vi "RunTest.vi"(8 "error in":errorcluster, 11 "Prueba31 in":refnum<class "Prueba03.lvclass">) -> (0 "error out":errorcluster, 2 "Resultado":string, 3 "Prueba31 out":refnum<class "Prueba03.lvclass">)   [LabVIEW 2019, in "Prueba03.lvclass"]
uses:
  Prueba03.lvclass
  Prueba03.lvclass/Prueba03.ctl
  <vilib>/Utility/miscctls.llb/LVRowAndColumnTypeDef.ctl
  QMH/Message Queue/Enqueue Message (Single).vi
  <vilib>/Utility/error.llb/Error Cluster From Error Code.vi
  RerenceAllControlsToolkit/_get control reference by name.vi
  <vilib>/ErrorRing/Error Ring.xnode
  QMH/Message Queue/Message Queue.lvlib
  QMH/User Event - Stop/User Event - Stop.lvlib
panel:
  in  "Tab":enum32{"externo", "interno"}(tab)
  out "Pict RingB_Ext":u16(ring)
  out "curva_referencia_Ext":dbl
  in  "cb_frec_Ext":string(combo)="63"
  in  "boton_generar_Ext":bool
  out "cumple_Ext":bool
  out "no_cumple_Ext":bool
  in  "seguir_Ext":bool
  out "voltaje_Ext":dbl format="%_3f"
  out "frecuencia_Ext":dbl format="%.2f"
  out "tipo generador_Ext":string
  out "Pict RingA_Ext":u16(ring)
  in  "Tabla_Ext":string[][](table)=[["63"], ["125"], ["250"], ["500"], ["1000"], ["2000"], ["4000"], ["8000"]]
  out "cumple_Int":bool
  out "no_cumple_Int":bool
  in  "seguir_Int":bool
  out "tipo generador_Int":string
  out "Pict RingA_Int":u16(ring)
  out "Pict RingB_Int":u16(ring)
  in  "Tabla_Int":string[][](table)
  # "Vienen de base de datos\nambos\ncambiar a numerico indicador"
  # "Cumple"
  # "No Cumple"
  # "Ponderación C"
  # "Curva de Referencia"
  # "Frecuencia"
  # "3. Ensayo con ponderación frecuencial C con señales acústicas. IEC 61672-3:2006 Cláusula 11"
  # "Monitoreo"
  # "Frecuencia"
  # "Hz"
  # "Voltaje"
  # "V"
  # "Cumple"
  # "No Cumple"
  # "Ponderación C"
  # "3. Ensayo con ponderación frecuencial C con señales acústicas. IEC 61672-3:2006 Cláusula 11"
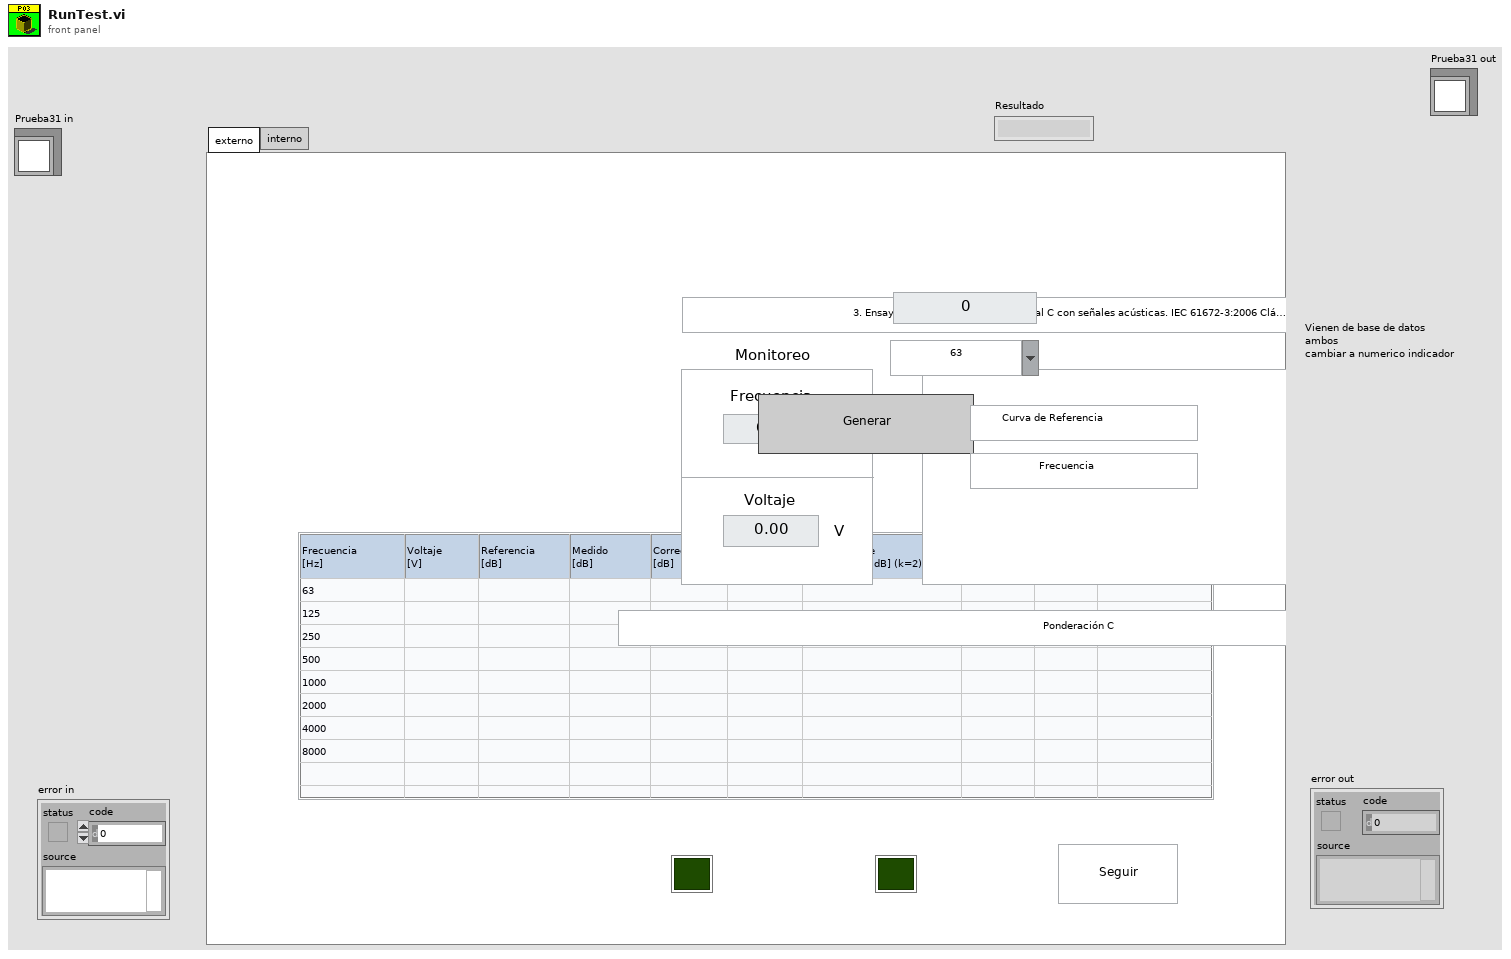
[diagram p1: front panel]
types:
  T1 = typedef "Message Queue.lvlib/All Message Queues.ctl" = cluster{"MHL":refnum<queue>, "Inst_CNT90":refnum<queue>, "Inst_DS360":refnum<queue>, "Inst_Keithley2002":refnum<queue>, "Inst_DAQ":refnum<queue>, "BD":refnum<queue>, "Pistofono":refnum<queue>, "Nexus":refnum<queue>}
  T2 = typedef "LVRowAndColumnTypeDef.ctl" = cluster{"Row":i32, "Column":i32}
  T3 = cluster{"ControlName":string, "ControlReference":refnum<vi>}[]
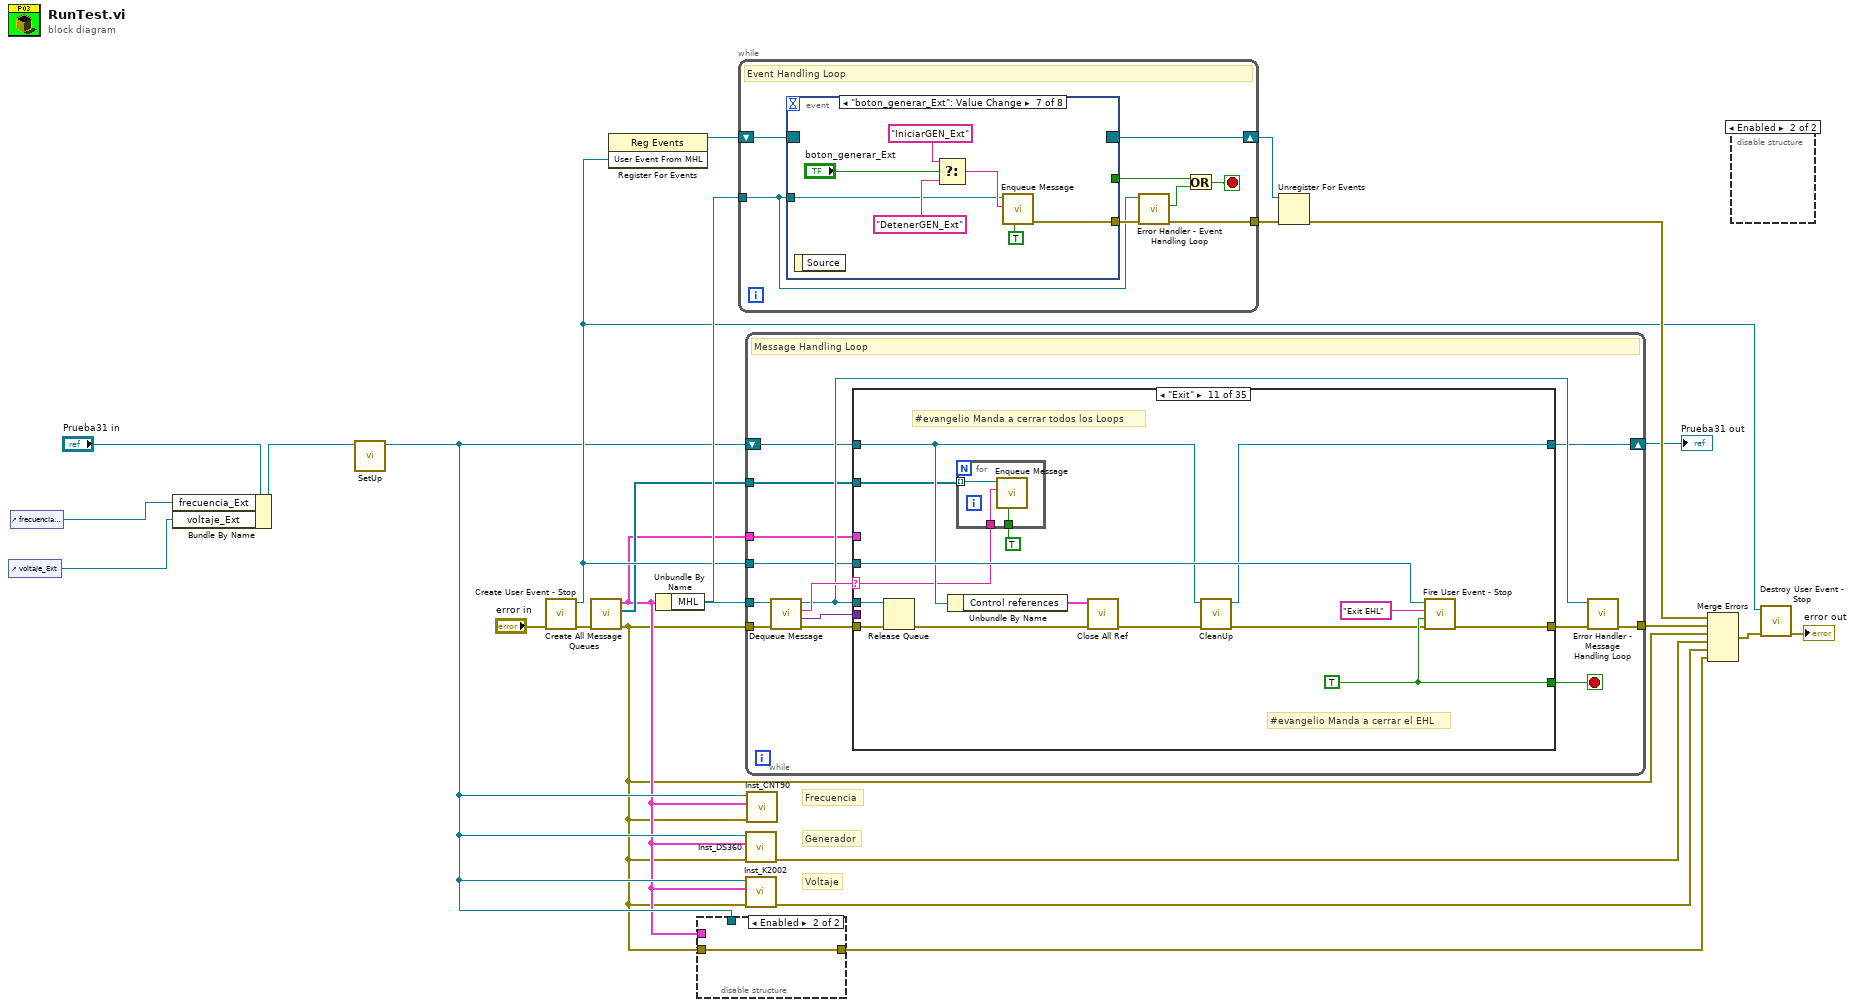
[diagram p0: block diagram]
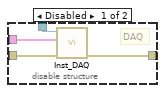
[diagram p2: hidden frame]
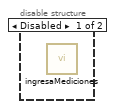
[diagram p3: hidden frame]
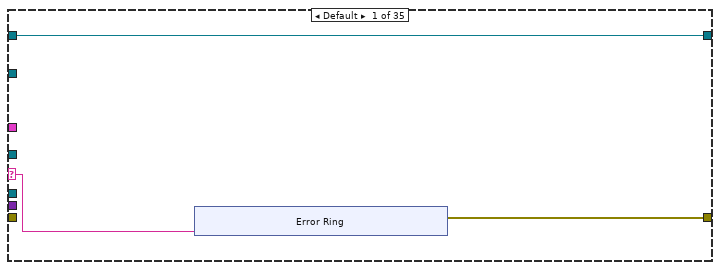
[diagram p4: hidden frame]
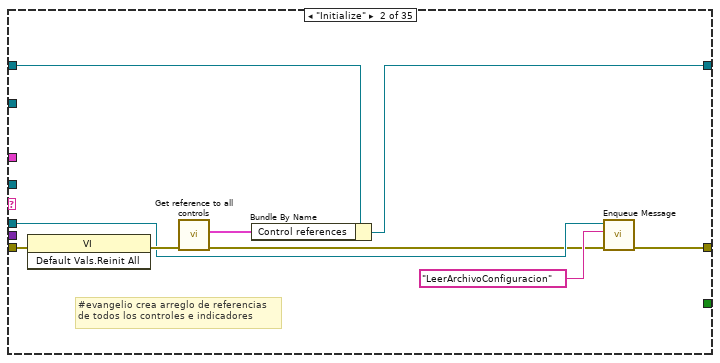
[diagram p5: hidden frame]
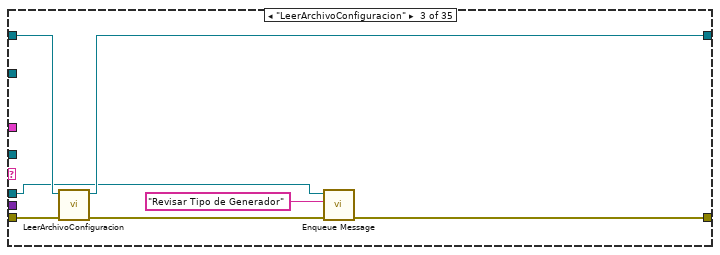
[diagram p6: hidden frame]
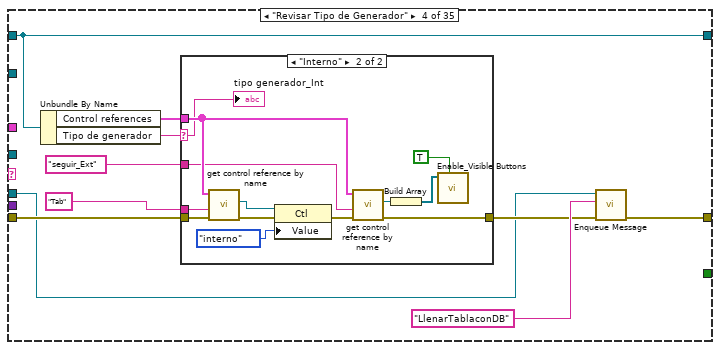
[diagram p7: hidden frame]
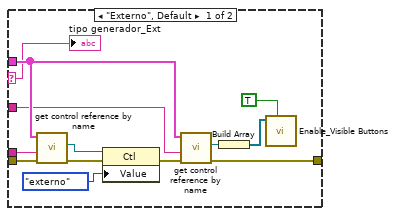
[diagram p8: hidden frame]
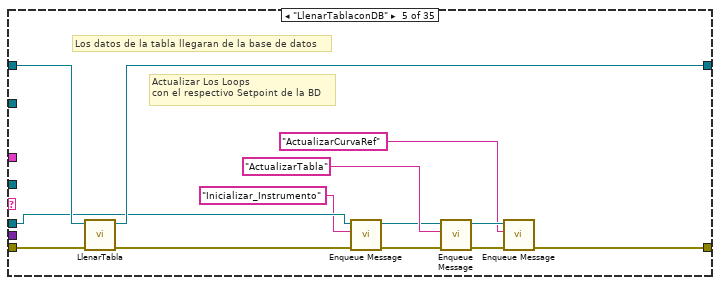
[diagram p9: hidden frame]
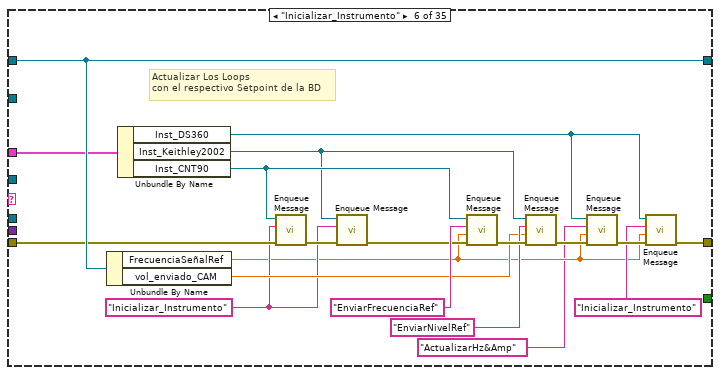
[diagram p10: hidden frame]
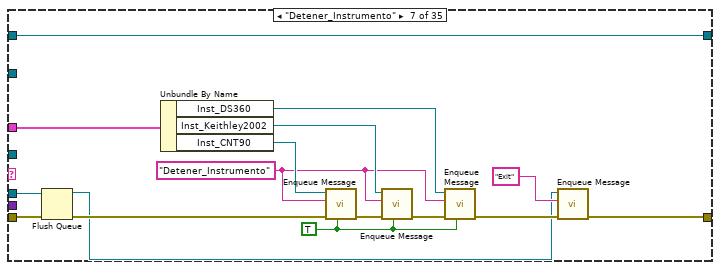
[diagram p11: hidden frame]
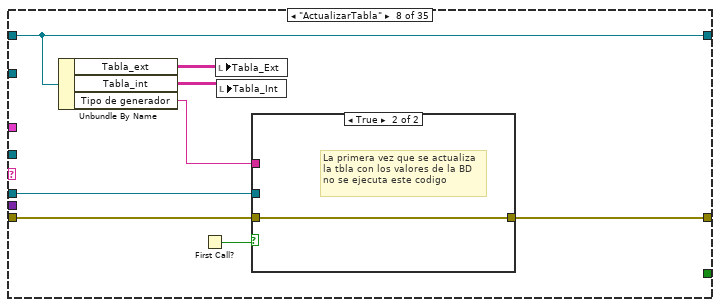
[diagram p12: hidden frame]
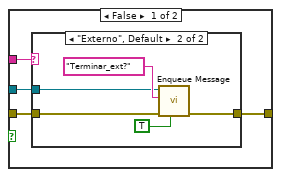
[diagram p13: hidden frame]
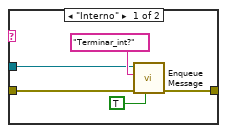
[diagram p14: hidden frame]
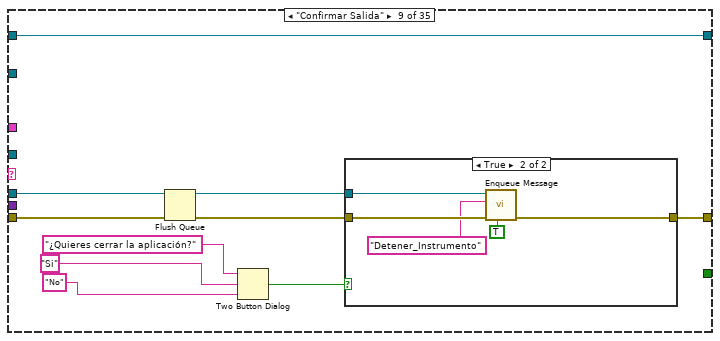
[diagram p15: hidden frame]
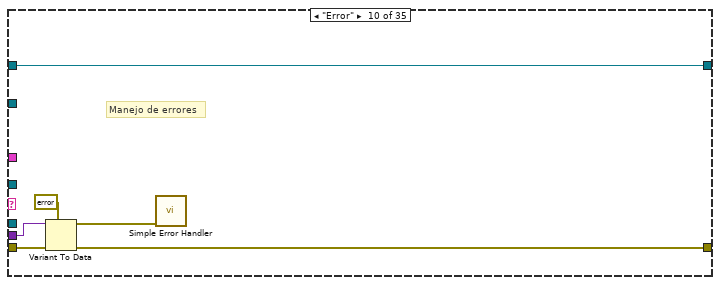
[diagram p17: hidden frame]
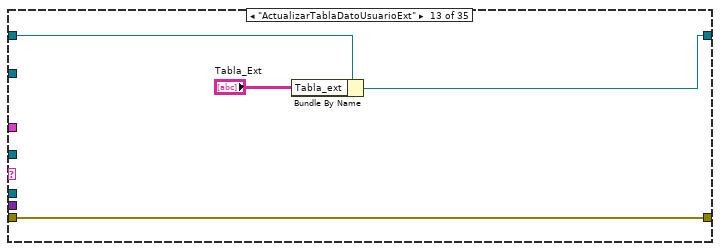
[diagram p19: hidden frame]
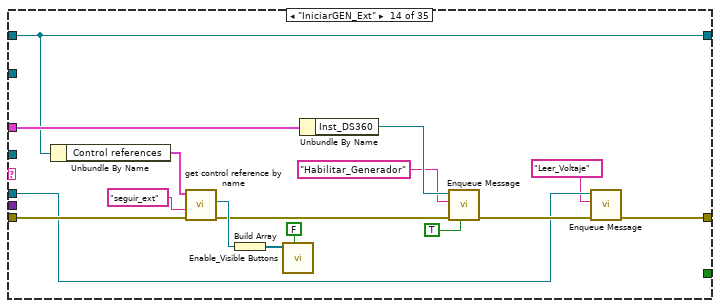
[diagram p20: hidden frame]
diagram:
  # "Voltaje"
  # "Generador"
  # "Frecuencia"
  n1 = control-ref of="voltaje_Ext"() -> (w1:refnum<vi>)
  n2 = control-ref of="frecuencia_Ext"() -> (w2:refnum<vi>)
  n3 = Bundle By Name(cluster="Prueba31 in", "frecuencia_Ext"=w2, "voltaje_Ext"=w1) -> (w3:refnum<class "Prueba03.lvclass">)
  n4 = call-dynamic "SetUp.vi"("Prueba03 in"=w3) -> ("Prueba03 out"=w6:refnum<class "Prueba03.lvclass">)  [unwired: 9 in, 1 out]
  n5 = call "Create User Event - Stop.vi"("error in (no error)"="error in") -> ("error out"=w20:errorcluster, "User Event From MHL"=w14:refnum<user-event>)  [unwired: 9 in]
  n6 = call "Create All Message Queues.vi"("error in (no error)"=w20) -> ("error out"=w4:errorcluster, "PL Queues Array"=w9:refnum<queue>[], "All Message Queues out"=w5:T1)  [unwired: 8 in]
  n7 = register-events(w14) -> (reference out=w23:refnum<event-registration>)  [unwired: 2 in, 1 out]
  n8 = Unbundle By Name(w5) -> ("MHL"=w19:refnum<queue>)
  n9 = disable-structure shown="Enabled" {
    disable-tunnel: w5 -> [w27 _]
    disable-tunnel: w4 -> [w26 w28]
    disable-tunnel: [w25 w28] -> w8
    disable-tunnel: w6 -> [w24 _]
    frame Disabled {
      # "DAQ"
      n10 = call "Inst_DAQ.vi"("error in"=w26, "All Message Queues in"=w27, "Prueba31 in"=w24) -> ("error out"=w25:errorcluster)  [unwired: 8 in]
    }
    frame Enabled {
    }
  }
  n11 = while {
    tunnel: w19 -> [w29]
    tunnel: [w33] -> w22
    shift-right: [w35] -> w21
    shift-left: w23 -> [w36]
    stop <- w30 stop-if-true
    # "Event Handling Loop"
    n12 = event shown="[6] \"boton_generar_Ext\": Value Change" {
      selector: w36 -> [_ _ _ _ _ _ _ _]
      dyn-events: [_ _ _ _ _ _ _ _] -> w35
      timeout: _ -> [_ _ _ _ _ _ _ _]
      tunnel: w29 -> [w39 _ w50 w53 w59 w63 w70 w77]
      tunnel: [w40 _ w47 w54 w61 w68 w75 w78] -> w34
      tunnel: [_ w41 _ _ _ _ _ _] -> w31
      event Panel Close? {
        w37 = TRUE
        n13 = event-data() -> ()  [unwired: 1 in, 1 out]
        n14 = call-poly "Enqueue Message.vi"("Priority Message? (F)"=w37, "Message"="Confirmar Salida", "Message Queue"=w39) -> ("error out"=w40:errorcluster)  [unwired: 7 in, 1 out]
        n15 = event-data("Discard?"=w37) -> ()  [unwired: 1 in, 1 out]
      }
      event User Event {
        n16 = event-data() -> ("User Event"=w43:string, "Event Data"=w42:variant)  [unwired: 1 in]
        n17 = case shown="\"Exit EHL\"" w43 {
          tunnel: w42 -> [_ w45]
          tunnel: [_ w44] -> w41
          frame Default {
          }
          frame "Exit EHL" {
            # "#evangelio Termina\nla ejecucion del EHL"
            n18 = Variant To Data(type=TRUE, Variant=w45) -> (data=w44:bool)  [unwired: 1 in, 1 out]
          }
        }
      }
      event "seguir_Ext": Value Change {
        n19 = event-data() -> ()  [unwired: 1 in, 1 out]
        n20 = call-poly "Enqueue Message.vi"("Priority Message? (F)"=TRUE, "Message"="Detener_Instrumento", "Message Queue"=w50) -> ("error out"=w47:errorcluster)  [unwired: 7 in, 1 out]
      }
      event "seguir_Int": Value Change {
        n21 = event-data() -> ()  [unwired: 1 in, 1 out]
        n22 = call-poly "Enqueue Message.vi"("Priority Message? (F)"=TRUE, "Message"="Exit", "Message Queue"=w53) -> ("error out"=w54:errorcluster)  [unwired: 7 in, 1 out]
      }
      event "Tabla_Ext": Value Change {
        n23 = event-data() -> ()  [unwired: 1 in, 1 out]
        n24 = property on="Tabla_Ext" class="Tbl (strict)"() -> ("Selection Start"=w55:T2)  [unwired: 2 in, 2 out]
        n25 = call-poly "Enqueue Message.vi"("Message"="ActualizarTablaDatoUsuarioExt", "Message Queue"=w59) -> ("error out"=w56:errorcluster, "dup Message Queue"=w58:refnum<queue>)  [unwired: 8 in]
        n26 = call-poly "Enqueue Message.vi"("error in (no error)"=w56, "Message Data"=w55, "Message"="Evaluacion_Ext", "Message Queue"=w58) -> ("error out"=w61:errorcluster)  [unwired: 6 in, 1 out]
      }
      event "Tabla_Int": Value Change {
        n27 = event-data() -> ()  [unwired: 1 in, 2 out]
        n28 = property on="Tabla_Int" class="Tbl (strict)"() -> ("Selection Start"=w66:T2)  [unwired: 2 in, 2 out]
        n29 = call-poly "Enqueue Message.vi"("Message"="ActualizarTablaDatoUsuarioInt", "Message Queue"=w63) -> ("error out"=w65:errorcluster, "dup Message Queue"=w64:refnum<queue>)  [unwired: 8 in]
        n30 = call-poly "Enqueue Message.vi"("error in (no error)"=w65, "Message Data"=w66, "Message"="Evaluacion_Int", "Message Queue"=w64) -> ("error out"=w68:errorcluster)  [unwired: 6 in, 1 out]
      }
      event "boton_generar_Ext": Value Change {
        n31 = event-data() -> ()  [unwired: 1 in, 1 out]
        n32 = Select(t="IniciarGEN_Ext" ("Message"), s="boton_generar_Ext", f="DetenerGEN_Ext" ("Message")) -> (s? t:f=w73:string)
        n33 = call-poly "Enqueue Message.vi"("Priority Message? (F)"=TRUE, "Message"=w73, "Message Queue"=w70) -> ("error out"=w75:errorcluster)  [unwired: 7 in, 1 out]
      }
      event "cb_frec_Ext": Value Change {
        (unwired) "ActualizarCurvaRef" ("Message")
        n34 = event-data() -> ()  [unwired: 1 in, 1 out]
        n35 = call-poly "Enqueue Message.vi"("Message"="NuevoValorFrecuencia", "Message Queue"=w77) -> ("error out"=w78:errorcluster)  [unwired: 8 in, 1 out]
      }
    }
    n36 = call "Error Handler - Event Handling Loop.vi"("error in (no error)"=w34, "Message Queue"=w29) -> ("dup error in"=w33:errorcluster, "Error?"=w32:bool)  [unwired: 7 in, 1 out]
    n37 = Or(x=w31, y=w32) -> (x .or. y?=w30:bool)
  }
  n38 = while {
    tunnel: w4 -> [w92]
    tunnel: w19 -> [w91]
    tunnel: [w85] -> w17
    shift-right: [w83] -> w15
    shift-left: w6 -> [w84]
    tunnel: w5 -> [w81]
    tunnel: w14 -> [w80]
    tunnel: w9 -> [w79]
    stop <- w82 stop-if-true
    # "Message Handling Loop"
    n39 = call "Dequeue Message.vi"("error in (no error)"=w92, "Message Queue"=w91) -> ("error out"=w88:errorcluster, "Message Data"=w89:variant, "Message"=w90:string, "dup Message Queue"=w87:refnum<queue>)  [unwired: 6 in]
    n40 = case shown="\"Exit\"" w90 {
      selector: w90 -> [w94 _ _ _ _ _ _ _ _ _ w249 _ _ _ _ _ _ _ _ _ w368 w377 _ _ _ _ _ _ _ _ _ _ _ _ _]
      tunnel: w87 -> [_ w106 w113 w119 w157 _ w190 w205 w226 _ w260 _ _ w272 w287 w297 w322 _ _ _ w363 _ w389 w406 _ w436 _ w458 w470 _ _ w484 w501 _ _]
      tunnel: w89 -> [_ _ _ _ _ _ _ _ _ w242 _ _ _ _ _ _ _ w337 w345 w348 w374 w384 w401 _ _ _ _ _ _ _ _ w496 _ _ _]
      tunnel: w88 -> [_ w111 w118 w125 w167 w178 w194 w206 w233 w243 w259 w266 w270 w279 w290 w300 w323 w338 w346 w349 w375 w385 w402 w415 w431 w440 w455 w465 w474 w477 w481 w497 w510 w529 w534]
      tunnel: [w93 w107 w114 w120 w160 w172 w189 w204 w232 w244 w257 w266 w270 w285 w289 w299 w314 w339 w347 w350 w372 w381 w393 w409 w431 w437 w451 w463 w473 w477 w481 w487 w504 w529 w534] -> w86
      tunnel: w84 -> [w95 w109 w117 w124 w166 w186 w201 w209 w234 w246 w250 w265 w268 w280 w294 w304 w328 w340 w343 w351 w376 w386 w397 w411 w427 w439 w454 w466 w475 w476 w479 w492 w506 w525 w533]
      tunnel: [w95 w108 w116 w124 w163 w186 w201 w209 w234 w246 w251 w265 w269 w280 w294 w304 w329 w340 w344 w351 w376 w386 w404 w411 w427 w439 w454 w461 w475 w476 w480 w499 w506 w525 w533] -> w83
      tunnel: [_ _ _ _ _ _ _ _ _ _ w254 _ _ _ _ _ _ _ _ _ _ _ _ _ _ _ _ _ _ _ _ _ _ _ _] -> w82
      tunnel: w81 -> [_ _ _ _ _ w184 w192 _ _ _ _ _ _ w286 w296 w306 w316 _ _ _ w371 w379 _ _ _ _ _ _ _ _ _ _ _ _ _]
      tunnel: w80 -> [_ _ _ _ _ _ _ _ _ _ w256 _ _ _ _ _ _ _ _ _ _ _ _ _ _ _ _ _ _ _ _ _ _ _ _]
      tunnel: w79 -> [_ _ _ _ _ _ _ _ _ _ w247 _ _ _ _ _ _ _ _ _ _ _ _ _ _ _ _ _ _ _ _ _ _ _ _]
      frame Default {
        n41 = xnode "Error Ring"("parameter 0"=w94) -> ("error out"=w93:errorcluster)
      }
      frame "Initialize" {
        # "#evangelio crea arreglo de referencias\nde todos los controles e indicadores"
        n42 = invoke class="VI" method="Default Vals.Reinit All"(error in=w111) -> (error out=w110:errorcluster)  [unwired: 2 in, 2 out]
        n43 = call "Get reference to all controls.vi"("error in (no error)"=w110) -> ("error out"=w103:errorcluster, "Control references"=w104:T3)  [unwired: 5 in]
        n44 = Bundle By Name(cluster=w109, "Control references"=w104) -> (w108:refnum<class "Prueba03.lvclass">)
        n45 = call-poly "Enqueue Message.vi"("error in (no error)"=w103, "Message"="LeerArchivoConfiguracion", "Message Queue"=w106) -> ("error out"=w107:errorcluster)  [unwired: 7 in, 1 out]
      }
      frame "LeerArchivoConfiguracion" {
        n46 = call "LeerArchivoConfiguracion.vi"("error in"=w118, "Prueba31 in"=w117) -> ("error out"=w115:errorcluster, "Prueba31 out"=w116:refnum<class "Prueba03.lvclass">)  [unwired: 8 in]
        n47 = call-poly "Enqueue Message.vi"("error in (no error)"=w115, "Message"="Revisar Tipo de Generador", "Message Queue"=w113) -> ("error out"=w114:errorcluster)  [unwired: 7 in, 1 out]
      }
      frame "Revisar Tipo de Generador" {
        n48 = Unbundle By Name(w124) -> ("Control references"=w127:T3, "Tipo de generador"=w128:string)
        n49 = case shown="\"Interno\"" w128 {
          selector: w128 -> [w129 w142]
          tunnel: w125 -> [w141 w154]
          tunnel: w127 -> [w136 w149]
          tunnel: "Tab" -> [w140 w153]
          tunnel: "seguir_Ext" -> [w134 w147]
          tunnel: [w131 w144] -> w121
          frame "Externo", Default {
            n50 = call-poly "get control reference by name.vi"("error in (no error)"=w141, "Control name"=w140, "Control references"=w136) -> ("error out"=w138:errorcluster, "Ctl Refnum"=w139:refnum<vi>)  [unwired: 3 in]
            n51 = property class="Ctl"(reference=w139, error in=w138, "Value"=enum32{"externo", "interno"}."externo" ("Tab Control")) -> (error out=w135:errorcluster)  [unwired: 1 out]
            n52 = call-poly "get control reference by name.vi"("error in (no error)"=w135, "Control name"=w134, "Control references"=w136) -> ("error out"=w131:errorcluster, "Ctl Refnum"=w133:refnum<vi>)  [unwired: 3 in]
            n53 = Build Array(w133) -> (w132:refnum<vi>[])
            n54 = call "Enable_Visible Buttons.vi"("Enable? (T)"=TRUE, "Controls Ref Array"=w132) -> ()  [unwired: 10 in]
            "tipo generador_Ext" <- w129
          }
          frame "Interno" {
            n55 = call-poly "get control reference by name.vi"("error in (no error)"=w154, "Control name"=w153, "Control references"=w149) -> ("error out"=w151:errorcluster, "Ctl Refnum"=w152:refnum<vi>)  [unwired: 3 in]
            n56 = property class="Ctl"(reference=w152, error in=w151, "Value"=enum32{"externo", "interno"}."interno" ("Tab Control")) -> (error out=w148:errorcluster)  [unwired: 1 out]
            n57 = call-poly "get control reference by name.vi"("error in (no error)"=w148, "Control name"=w147, "Control references"=w149) -> ("error out"=w144:errorcluster, "Ctl Refnum"=w146:refnum<vi>)  [unwired: 3 in]
            n58 = Build Array(w146) -> (w145:refnum<vi>[])
            n59 = call "Enable_Visible Buttons.vi"("Enable? (T)"=TRUE, "Controls Ref Array"=w145) -> ()  [unwired: 10 in]
            "tipo generador_Int" <- w142
          }
        }
        n60 = call-poly "Enqueue Message.vi"("error in (no error)"=w121, "Message"="LlenarTablaconDB", "Message Queue"=w119) -> ("error out"=w120:errorcluster)  [unwired: 7 in, 1 out]
      }
      frame "LlenarTablaconDB" {
        # "Actualizar Los Loops\ncon el respectivo Setpoint de la BD"
        # "Los datos de la tabla llegaran de la base de datos"
        n61 = call "LlenarTabla.vi"("error in (no error)"=w167, "Prueba32 in"=w166) -> ("error out"=w165:errorcluster, "Prueba32 out"=w163:refnum<class "Prueba03.lvclass">)  [unwired: 8 in]
        n62 = call-poly "Enqueue Message.vi"("error in (no error)"=w165, "Message"="Inicializar_Instrumento", "Message Queue"=w157) -> ("error out"=w158:errorcluster, "dup Message Queue"=w156:refnum<queue>)  [unwired: 7 in]
        n63 = call-poly "Enqueue Message.vi"("error in (no error)"=w158, "Message"="ActualizarTabla", "Message Queue"=w156) -> ("error out"=w161:errorcluster, "dup Message Queue"=w162:refnum<queue>)  [unwired: 7 in]
        n64 = call-poly "Enqueue Message.vi"("error in (no error)"=w161, "Message"="ActualizarCurvaRef", "Message Queue"=w162) -> ("error out"=w160:errorcluster)  [unwired: 7 in, 1 out]
      }
      frame "Inicializar_Instrumento" {
        w174 = "Inicializar_Instrumento" ("Message")
        # "Actualizar Los Loops\ncon el respectivo Setpoint de la BD"
        n65 = Unbundle By Name(w186) -> ("FrecuenciaSeñalRef"=w169:dbl, "vol_enviado_CAM"=w181:dbl)
        n66 = Unbundle By Name(w184) -> ("Inst_DS360"=w171:refnum<queue>, "Inst_Keithley2002"=w175:refnum<queue>, "Inst_CNT90"=w179:refnum<queue>)
        n67 = call-poly "Enqueue Message.vi"("error in (no error)"=w178, "Message"=w174, "Message Queue"=w179) -> ("error out"=w177:errorcluster)  [unwired: 7 in, 1 out]
        n68 = call-poly "Enqueue Message.vi"("error in (no error)"=w177, "Message"=w174, "Message Queue"=w175) -> ("error out"=w176:errorcluster)  [unwired: 7 in, 1 out]
        n69 = call-poly "Enqueue Message.vi"("error in (no error)"=w176, "Message Data"=w169, "Message"="EnviarFrecuenciaRef", "Message Queue"=w179) -> ("error out"=w185:errorcluster)  [unwired: 6 in, 1 out]
        n70 = call-poly "Enqueue Message.vi"("error in (no error)"=w185, "Message Data"=w181, "Message"="EnviarNivelRef", "Message Queue"=w175) -> ("error out"=w180:errorcluster)  [unwired: 6 in, 1 out]
        n71 = call-poly "Enqueue Message.vi"("error in (no error)"=w180, "Message Data"=w169, "Message"="ActualizarHz&Amp", "Message Queue"=w171) -> ("error out"=w173:errorcluster)  [unwired: 6 in, 1 out]
        n72 = call-poly "Enqueue Message.vi"("error in (no error)"=w173, "Message Data"=w169, "Message"="Inicializar_Instrumento", "Message Queue"=w171) -> ("error out"=w172:errorcluster)  [unwired: 6 in, 1 out]
      }
      frame "Detener_Instrumento" {
        w195 = TRUE ("Priority Message? (F)")
        w196 = "Detener_Instrumento" ("Message")
        n73 = Flush Queue(queue=w190, error in (no error)=w194) -> (queue out=w187:refnum<queue>, error out=w191:errorcluster)  [unwired: 1 out]
        n74 = Unbundle By Name(w192) -> ("Inst_DS360"=w197:refnum<queue>, "Inst_Keithley2002"=w198:refnum<queue>, "Inst_CNT90"=w200:refnum<queue>)
        n75 = call-poly "Enqueue Message.vi"("Priority Message? (F)"=w195, "error in (no error)"=w191, "Message"=w196, "Message Queue"=w200) -> ("error out"=w199:errorcluster)  [unwired: 6 in, 1 out]
        n76 = call-poly "Enqueue Message.vi"("Priority Message? (F)"=w195, "error in (no error)"=w199, "Message"=w196, "Message Queue"=w198) -> ("error out"=w193:errorcluster)  [unwired: 6 in, 1 out]
        n77 = call-poly "Enqueue Message.vi"("Priority Message? (F)"=w195, "Message"=w196, "Message Queue"=w197) -> ()  [unwired: 7 in, 2 out]
        n78 = call-poly "Enqueue Message.vi"("error in (no error)"=w193, "Message"="Exit", "Message Queue"=w187) -> ("error out"=w189:errorcluster)  [unwired: 7 in, 1 out]
      }
      frame "ActualizarTabla" {
        n79 = Unbundle By Name(w209) -> ("Tabla_ext"=w208:string[][], "Tabla_int"=w207:string[][], "Tipo de generador"=w203:string)
        n80 = First Call?() -> (First Call?: T/F=w202:bool)
        n81 = local write "Tabla_Ext"(w208) -> ()
        n82 = local write "Tabla_Int"(w207) -> ()
        n83 = case shown="True" w202 {
          tunnel: w206 -> [w213 w224]
          tunnel: w205 -> [w212 _]
          tunnel: [w211 w224] -> w204
          tunnel: w203 -> [w210 _]
          frame False {
            n84 = case shown="\"Externo\", Default" w210 {
              tunnel: w213 -> [w216 w222]
              tunnel: w212 -> [w217 w221]
              tunnel: [w215 w220] -> w211
              frame "Interno" {
                n85 = call-poly "Enqueue Message.vi"("Priority Message? (F)"=TRUE, "error in (no error)"=w216, "Message"="Terminar_int?", "Message Queue"=w217) -> ("error out"=w215:errorcluster)  [unwired: 6 in, 1 out]
              }
              frame "Externo", Default {
                n86 = call-poly "Enqueue Message.vi"("Priority Message? (F)"=TRUE, "error in (no error)"=w222, "Message"="Terminar_ext?", "Message Queue"=w221) -> ("error out"=w220:errorcluster)  [unwired: 6 in, 1 out]
              }
            }
          }
          frame True {
            # "La primera vez que se actualiza\nla tbla con los valores de la BD\nno se ejecuta este codigo"
          }
        }
      }
      frame "Confirmar Salida" {
        n87 = Flush Queue(queue=w226, error in (no error)=w233) -> (queue out=w225:refnum<queue>, error out=w227:errorcluster)  [unwired: 1 out]
        n88 = Two Button Dialog(message="¿Quieres cerrar la aplicación?", 1:"No" ("T button name (\"OK\")"), 2:"Si" ("T button name (\"OK\")")) -> (T button?=w228:bool)
        n89 = case shown="True" w228 {
          tunnel: w227 -> [w235 w240]
          tunnel: [w235 w237] -> w232
          tunnel: w225 -> [_ w238]
          frame False {
          }
          frame True {
            n90 = call-poly "Enqueue Message.vi"("Priority Message? (F)"=TRUE, "error in (no error)"=w240, "Message"="Detener_Instrumento", "Message Queue"=w238) -> ("error out"=w237:errorcluster)  [unwired: 6 in, 1 out]
          }
        }
      }
      frame "Error" {
        # "Manejo de errores"
        n91 = Variant To Data(error in=w243, type=errorcluster {"status"=FALSE, "code"=0, "source"=""} ("error constant"), Variant=w242) -> (data=w241:errorcluster, error out=w244:errorcluster)
        n92 = call <vilib>:"Simple Error Handler.vi"("error in (no error)"=w241) -> ()  [unwired: 4 in, 5 out]
      }
      frame "Exit" {
        w254 = TRUE
        # "#evangelio Manda a cerrar el EHL"
        # "#evangelio Manda a cerrar todos los Loops"
        n93 = Release Queue(queue=w260, error in (no error)=w259) -> (error out=w258:errorcluster)  [unwired: 1 in, 2 out]
        n94 = Unbundle By Name(w250) -> ("Control references"=w261:T3)
        n95 = for {
          tunnel: w247 -> [w264] mode=indexing
          tunnel: w249 -> [w263]
          tunnel: TRUE -> [w262]
          n96 = call-poly "Enqueue Message.vi"("Priority Message? (F)"=w262, "Message"=w263, "Message Queue"=w264) -> ()  [unwired: 7 in, 2 out]
        }
        n97 = call "Close All Ref.vi"("error in (no error)"=w258, "Control references"=w261) -> ("error out"=w253:errorcluster)  [unwired: 9 in]
        n98 = call-dynamic "CleanUp.vi"("error in (no error)"=w253, "Prueba03 in"=w250) -> ("error out"=w252:errorcluster, "Prueba03 out"=w251:refnum<class "Prueba03.lvclass">)  [unwired: 8 in]
        n99 = call "Fire User Event - Stop.vi"("error in (no error)"=w252, "Event Data"=w254, "User Event"="Exit EHL", "User Event in"=w256) -> ("error out"=w257:errorcluster)  [unwired: 7 in]
      }
      frame "---- EXT ----" {
      }
      frame "ActualizarTablaDatoUsuarioExt" {
        n100 = Bundle By Name(cluster=w268, "Tabla_ext"="Tabla_Ext") -> (w269:refnum<class "Prueba03.lvclass">)
      }
      frame "IniciarGEN_Ext" {
        n101 = Unbundle By Name(w280) -> ("Control references"=w281:T3)
        n102 = call-poly "get control reference by name.vi"("error in (no error)"=w279, "Control name"="seguir_ext", "Control references"=w281) -> ("error out"=w275:errorcluster, "Ctl Refnum"=w283:refnum<vi>)  [unwired: 3 in]
        n103 = Build Array(w283) -> (w282:refnum<vi>[])
        n104 = call "Enable_Visible Buttons.vi"("Enable? (T)"=FALSE, "Controls Ref Array"=w282) -> ()  [unwired: 10 in]
        n105 = Unbundle By Name(w286) -> ("Inst_DS360"=w277:refnum<queue>)
        n106 = call-poly "Enqueue Message.vi"("Priority Message? (F)"=TRUE, "error in (no error)"=w275, "Message"="Habilitar_Generador", "Message Queue"=w277) -> ("error out"=w274:errorcluster)  [unwired: 6 in, 1 out]
        n107 = call-poly "Enqueue Message.vi"("error in (no error)"=w274, "Message"="Leer_Voltaje", "Message Queue"=w272) -> ("error out"=w285:errorcluster)  [unwired: 7 in, 1 out]
      }
      frame "Leer_Voltaje" {
        n108 = call-poly "Enqueue Message.vi"("error in (no error)"=w290, "Message"="Leer_Frecuencia", "Message Queue"=w287) -> ("error out"=w295:errorcluster)  [unwired: 7 in, 1 out]
        n109 = Unbundle By Name(w296) -> ("Inst_Keithley2002"=w293:refnum<queue>)
        n110 = call-poly "Enqueue Message.vi"("Message"="Leer_Instrumento", "Message Queue"=w293) -> ()  [unwired: 8 in, 2 out]
        n111 = call "Time Delay"("error in (no error)"=w295, "Delay Time (s)"=1.0) -> ("error out"=w289:errorcluster)  [unwired: 9 in]
      }
      frame "Leer_Frecuencia" {
        n112 = call-poly "Enqueue Message.vi"("error in (no error)"=w300, "Message"="Leer_Voltaje", "Message Queue"=w297) -> ("error out"=w305:errorcluster)  [unwired: 7 in, 1 out]
        n113 = Unbundle By Name(w306) -> ("Inst_CNT90"=w303:refnum<queue>)
        n114 = call-poly "Enqueue Message.vi"("Message"="Leer_Instrumento", "Message Queue"=w303) -> ()  [unwired: 8 in, 2 out]
        n115 = call "Time Delay2"("error in (no error)"=w305, "Delay Time (s)"=1.0) -> ("error out"=w299:errorcluster)  [unwired: 9 in]
      }
      frame "DetenerGEN_Ext" {
        w309 = 0.0 ("frecuencia_Ext")
        w321 = 0.0 ("frecuencia_Ext")
        n116 = Unbundle By Name(w328) -> ("Tabla_ext"=w327:string[][], "voltMedido"=w312:dbl, "Control references"=w331:T3)
        n117 = Flush Queue(queue=w322, error in (no error)=w323) -> (queue out=w319:refnum<queue>, error out=w324:errorcluster)  [unwired: 1 out]
        n118 = local write "frecuencia_Ext"(w321) -> ()
        n119 = local write "voltaje_Ext"(w321) -> ()
        n120 = call-poly "get control reference by name.vi"("error in (no error)"=w324, "Control name"="seguir_ext", "Control references"=w331) -> ("error out"=w320:errorcluster, "Ctl Refnum"=w333:refnum<vi>)  [unwired: 3 in]
        n121 = Build Array(w333) -> (w332:refnum<vi>[])
        n122 = Number To Fractional String(use system decimal point (T)=TRUE, number=w312, precision (6)=i16 3) -> (F-format string=w325:string)  [unwired: 1 in]
        n123 = call "Enable_Visible Buttons.vi"("Controls Ref Array"=w332) -> ()  [unwired: 11 in]
        n124 = Unbundle By Name(w316) -> ("Inst_DS360"=w315:refnum<queue>, "Inst_Keithley2002"=w311:refnum<queue>)
        n125 = call "LlenarVoltajeTabla.vi"("Frecuencia"="cb_frec_Ext", "Dato"=w325, "Tabla in"=w327) -> ("Tabla out"=w317:string[][])  [unwired: 8 in]
        n126 = call-poly "Enqueue Message.vi"("error in (no error)"=w320, "Message"="SiguienteFrecuencia" ("Control name"), "Message Queue"=w319) -> ("error out"=w308:errorcluster)  [unwired: 7 in, 1 out]
        n127 = Bundle By Name(cluster=w328, "Tabla_ext"=w317) -> (w329:refnum<class "Prueba03.lvclass">)
        n128 = Flush Queue(queue=w311, error in (no error)=w308) -> (error out=w310:errorcluster)  [unwired: 2 out]
        n129 = local write "Tabla_Ext"(w317) -> ()
        n130 = call-poly "Enqueue Message.vi"("error in (no error)"=w310, "Message"="Dehabilitar_Generador", "Message Queue"=w315) -> ("error out"=w314:errorcluster)  [unwired: 7 in, 1 out]
        n131 = local write "frecuencia_Ext"(w309) -> ()
        n132 = local write "voltaje_Ext"(w309) -> ()
      }
      frame "DatoRecibidoCNT90" {
        n133 = Variant To Data(error in=w338, type=0.0, Variant=w337) -> (data=→"frecuencia_Ext":dbl, error out=w339:errorcluster)
      }
      frame "DatoRecibidoK2002" {
        n134 = Variant To Data(error in=w346, type=0.0, Variant=w345) -> (data=w341:dbl, error out=w347:errorcluster)
        "voltaje_Ext" <- w341
        n135 = Bundle By Name(cluster=w343, "voltMedido"=w341) -> (w344:refnum<class "Prueba03.lvclass">)
      }
      frame "DatoRecibidoDS360" {
        n136 = disable-structure shown="Disabled" {
          disable-tunnel: [w354 w355] -> w350
          disable-tunnel: w349 -> [w353 w355]
          disable-tunnel: w348 -> [w352 _]
          frame Disabled {
            n137 = Variant To Data(error in=w353, Variant=w352) -> (error out=w354:errorcluster)  [unwired: 1 in, 1 out]
          }
          frame Enabled {
          }
        }
      }
      frame "EnviarFrecuenciaRef" {
        w359 = 0.0 ("frecuencia_Ext")
        w367 = TRUE ("Priority Message? (F)")
        # "envía frecuencia al generador"
        n138 = Flush Queue(queue=w363, error in (no error)=w375) -> (error out=w364:errorcluster)  [unwired: 2 out]
        n139 = Variant To Data(error in=w364, type=w368, Variant=w374) -> (data=w373:string, error out=w358:errorcluster)
        n140 = Unbundle By Name(w371) -> ("Inst_Keithley2002"=w360:refnum<queue>, "Inst_DS360"=w369:refnum<queue>, "Inst_CNT90"=w370:refnum<queue>)
        n141 = Fract/Exp String To Number(string=w373) -> (number=w365:dbl)  [unwired: 3 in, 1 out]
        n142 = Flush Queue(queue=w370, error in (no error)=w358) -> (queue out=w361:refnum<queue>, error out=w357:errorcluster)  [unwired: 1 out]
        n143 = Flush Queue(queue=w360, error in (no error)=w357) -> (error out=w356:errorcluster)  [unwired: 2 out]
        n144 = Flush Queue(queue=w369) -> (queue out=w362:refnum<queue>)  [unwired: 1 in, 2 out]
        n145 = call-poly "Enqueue Message.vi"("Priority Message? (F)"=w367, "error in (no error)"=w356, "Message Data"=w365, "Message"=w368, "Message Queue"=w361) -> ("error out"=w372:errorcluster)  [unwired: 5 in, 1 out]
        n146 = local write "frecuencia_Ext"(w359) -> ()
        n147 = local write "voltaje_Ext"(w359) -> ()
        n148 = call-poly "Enqueue Message.vi"("Priority Message? (F)"=w367, "Message Data"=w365, "Message"="ActualizarHz&Amp", "Message Queue"=w362) -> ()  [unwired: 6 in, 2 out]
      }
      frame "EnviarNivelRef" {
        n149 = Variant To Data(error in=w385, type=w377, Variant=w384) -> (data=w383:string, error out=w382:errorcluster)
        n150 = Unbundle By Name(w379) -> ("Inst_Keithley2002"=w378:refnum<queue>)
        n151 = Fract/Exp String To Number(string=w383) -> (number=w380:dbl)  [unwired: 3 in, 1 out]
        n152 = call-poly "Enqueue Message.vi"("error in (no error)"=w382, "Message Data"=w380, "Message"=w377, "Message Queue"=w378) -> ("error out"=w381:errorcluster)  [unwired: 6 in, 1 out]
      }
      frame "Evaluacion_Ext" {
        # "columna"
        n153 = Variant To Data(error in=w402, type=T2 {"Row"=0, "Column"=0} ("Selection Start"), Variant=w401) -> (data=w399:T2, error out=w403:errorcluster)
        n154 = Unbundle By Name(w399) -> ("Row"=w396:i32)  [unwired: 1 out]
        n155 = call "ObtenerDatosdelatabla.vi"("tipo_gen"="externo", "Column"=3, "Row"=w396, "Prueba32 in"=w397) -> ("Prueba32 out"=w398:refnum<class "Prueba03.lvclass">)  [unwired: 7 in]
        n156 = call "cumplimiento_ext.vi"("error in (no error)"=w403, "Prueba08 in"=w398) -> ("error out"=w395:errorcluster, "Prueba08 out"=w404:refnum<class "Prueba03.lvclass">)  [unwired: 7 in, 1 out]
        n157 = Flush Queue(queue=w389, error in (no error)=w395) -> (queue out=w388:refnum<queue>, error out=w390:errorcluster)  [unwired: 1 out]
        n158 = call-poly "Enqueue Message.vi"("Priority Message? (F)"=TRUE, "error in (no error)"=w390, "Message"="ActualizarTabla", "Message Queue"=w388) -> ("error out"=w393:errorcluster)  [unwired: 6 in, 1 out]
      }
      frame "Terminar_ext?" {
        # "si son todos\ndistntos a cero\nentonces todos se\nhan evaluado"
        n159 = Unbundle By Name(w411) -> ("Tabla_ext"=w410:string[][])
        n160 = Index Array(array=w410, index (col)=9 ("disabled index (col)")) -> (element=w413:string[])  [unwired: 1 in]
        n161 = Flush Queue(queue=w406, error in (no error)=w415) -> (queue out=w405:refnum<queue>, error out=w407:errorcluster)  [unwired: 1 out]
        n162 = for {
          tunnel: [w423] -> w412 mode=indexing
          tunnel: w413 -> [w421] mode=indexing
          n163 = Not Equal?(x=w421, y="--") -> (x != y?=w423:bool)
        }
        n164 = And Array Elements(Boolean array=w412) -> (logical AND=w408:bool)
        n165 = case shown="False" w408 {
          tunnel: w407 -> [w416 w420]
          tunnel: [w416 w419] -> w409
          tunnel: w405 -> [_ w418]
          frame False {
          }
          frame True {
            n166 = call-poly "Enqueue Message.vi"("error in (no error)"=w420, "Message"="Cumple_ext?", "Message Queue"=w418) -> ("error out"=w419:errorcluster)  [unwired: 7 in, 1 out]
          }
        }
      }
      frame "Cumple_ext?" {
        # "si todos cumplen\nentonces el ensayo\ncumple"
        n167 = Unbundle By Name(w427) -> ("Tabla_ext"=w426:string[][])
        n168 = Index Array(array=w426, index (col)=9 ("disabled index (col)")) -> (element=w429:string[])  [unwired: 1 in]
        n169 = for {
          tunnel: [w434] -> w428 mode=indexing
          tunnel: w429 -> [w432] mode=indexing
          n170 = Equal?(x=w432, y="Cumple") -> (x = y?=w434:bool)
        }
        n171 = And Array Elements(Boolean array=w428) -> (logical AND=w424:bool)
        "cumple_Ext" <- w424
        n172 = Not(x=w424) -> (.not. x?=→"no_cumple_Ext":bool)
      }
      frame "ActualizarCurvaRef" {
        n173 = disable-structure shown="Enabled" {
          disable-tunnel: w439 -> [w447 w449]
          disable-tunnel: [w441 w448] -> w438
          frame Disabled {
            n174 = Unbundle By Name(w447) -> ("Tabla_ext"=w445:string[][])
            n175 = local read "cb_frec_Ext"() -> (w446:string)
            n176 = call "ObtenerFilaEnUso.vi"("Tabla in"=w445, "Frecuencia"=w446) -> ("index of element"=w444:i32)  [unwired: 9 in]
            n177 = Index Array(array=w445, index (row)=w444, index (col)=1 ("disabled index (col)")) -> (element=w442:string)
            n178 = Fract/Exp String To Number(string=w442) -> (number=w441:dbl)  [unwired: 3 in, 1 out]
          }
          frame Enabled {
            n179 = Unbundle By Name(w449) -> ("NivelSeñalRef"=w448:dbl)
          }
        }
        "curva_referencia_Ext" <- w438
        n180 = call-poly "Enqueue Message.vi"("error in (no error)"=w440, "Message"="ActualizarComboBoxFrecuenciaExt", "Message Queue"=w436) -> ("error out"=w437:errorcluster)  [unwired: 7 in, 1 out]
      }
      frame "ActualizarComboBoxFrecuenciaExt" {
        n181 = Unbundle By Name(w454) -> ("Frecuencias(Hz)"=w453:string[])
        n182 = Index Array(array=w453, index=0) -> (element=w450:string)
        n183 = property on="cb_frec_Ext" class="CmbBox"(error in=w455, "Value"=w450) -> (error out=w451:errorcluster)  [unwired: 1 in, 1 out]
      }
      frame "SiguienteFrecuencia" {
        w456 = 0.0 ("frecuencia_Ext")
        n184 = Flush Queue(queue=w458, error in (no error)=w465) -> (queue out=w457:refnum<queue>, error out=w459:errorcluster)  [unwired: 1 out]
        n185 = call "NuevaFrecuencia.vi"("error in (no error)"=w459, "Prueba031 in"=w466) -> ("error out"=w464:errorcluster, "newFrec"=w460:string, "Prueba031 out"=w461:refnum<class "Prueba03.lvclass">)  [unwired: 7 in]
        n186 = call-poly "Enqueue Message.vi"("error in (no error)"=w464, "Message Data"=w460, "Message"="EnviarFrecuenciaRef", "Message Queue"=w457) -> ("error out"=w463:errorcluster)  [unwired: 6 in, 1 out]
        n187 = local write "frecuencia_Ext"(w456) -> ()
        n188 = local write "voltaje_Ext"(w456) -> ()
      }
      frame "NuevoValorFrecuencia" {
        n189 = Flush Queue(queue=w470, error in (no error)=w474) -> (queue out=w469:refnum<queue>, error out=w471:errorcluster)  [unwired: 1 out]
        n190 = property on="cb_frec_Ext" class="CmbBox"(error in=w471) -> (error out=w468:errorcluster, "Value"=w467:string)  [unwired: 1 in, 1 out]
        n191 = call-poly "Enqueue Message.vi"("error in (no error)"=w468, "Message Data"=w467, "Message"="EnviarFrecuenciaRef", "Message Queue"=w469) -> ("error out"=w473:errorcluster)  [unwired: 6 in, 1 out]
      }
      frame "---- INT ----" {
      }
      frame "ActualizarTablaDatoUsuarioInt" {
        n192 = Bundle By Name(cluster=w479, "Tabla_int"="Tabla_Int") -> (w480:refnum<class "Prueba03.lvclass">)
      }
      frame "Evaluacion_Int" {
        n193 = Variant To Data(error in=w497, type=T2 {"Row"=0, "Column"=0} ("Selection Start"), Variant=w496) -> (data=w494:T2, error out=w498:errorcluster)
        n194 = Unbundle By Name(w494) -> ("Row"=w491:i32)  [unwired: 1 out]
        n195 = call "ObtenerDatosdelatabla.vi"("tipo_gen"="interno", "Column"=2, "Row"=w491, "Prueba32 in"=w492) -> ("Prueba32 out"=w493:refnum<class "Prueba03.lvclass">)  [unwired: 7 in]
        n196 = call "cumplimiento_int.vi"("error in (no error)"=w498, "Prueba08 in"=w493) -> ("error out"=w490:errorcluster, "Prueba08 out"=w499:refnum<class "Prueba03.lvclass">)  [unwired: 7 in, 1 out]
        n197 = Flush Queue(queue=w484, error in (no error)=w490) -> (queue out=w483:refnum<queue>, error out=w485:errorcluster)  [unwired: 1 out]
        n198 = call-poly "Enqueue Message.vi"("Priority Message? (F)"=TRUE, "error in (no error)"=w485, "Message"="ActualizarTabla", "Message Queue"=w483) -> ("error out"=w487:errorcluster)  [unwired: 6 in, 1 out]
      }
      frame "Terminar_int?" {
        # "si son todos\ndistntos a cero\nentonces todos se\nhan evaluado"
        n199 = Unbundle By Name(w506) -> ("Tabla_int"=w505:string[][])
        n200 = Index Array(array=w505, index (col)=8 ("disabled index (col)")) -> (element=w508:string[])  [unwired: 1 in]
        n201 = Flush Queue(queue=w501, error in (no error)=w510) -> (queue out=w500:refnum<queue>, error out=w502:errorcluster)  [unwired: 1 out]
        n202 = for {
          tunnel: [w518] -> w507 mode=indexing
          tunnel: w508 -> [w516] mode=indexing
          n203 = Not Equal?(x=w516, y="--") -> (x != y?=w518:bool)
        }
        n204 = And Array Elements(Boolean array=w507) -> (logical AND=w503:bool)
        n205 = case shown="False" w503 {
          tunnel: w502 -> [w511 w515]
          tunnel: [w511 w514] -> w504
          tunnel: w500 -> [_ w513]
          frame False {
          }
          frame True {
            n206 = call-poly "Enqueue Message.vi"("error in (no error)"=w515, "Message"="Cumple_int?", "Message Queue"=w513) -> ("error out"=w514:errorcluster)  [unwired: 7 in, 1 out]
          }
        }
      }
      frame "Cumple_int?" {
        # "si todos cumplen\nentonces el ensayo\ncumple"
        n207 = Unbundle By Name(w525) -> ("Tabla_int"=w524:string[][])
        n208 = Index Array(array=w524, index (col)=8 ("disabled index (col)")) -> (element=w527:string[])  [unwired: 1 in]
        n209 = for {
          tunnel: [w532] -> w526 mode=indexing
          tunnel: w527 -> [w530] mode=indexing
          n210 = Equal?(x=w530, y="Cumple") -> (x = y?=w532:bool)
        }
        n211 = And Array Elements(Boolean array=w526) -> (logical AND=w522:bool)
        "cumple_Int" <- w522
        n212 = Not(x=w522) -> (.not. x?=→"no_cumple_Int":bool)
        n213 = Select(t="Cumple" ("y"), s=w522, f="No Cumple" ("y")) -> (s? t:f=→"Resultado":string)
      }
      frame "--------------------------Contoles---------------------------" {
      }
    }
    n214 = call "Error Handler - Message Handling Loop.vi"("error in (no error)"=w86, "Message Queue"=w87) -> ("dup error in"=w85:errorcluster)  [unwired: 8 in, 1 out]
  }
  "Prueba31 out" <- w15
  n215 = call "Inst_DS360.vi"("error in"=w4, "All Message Queues in"=w5, "Prueba31 in"=w6) -> ("error out"=w11:errorcluster)  [unwired: 8 in]
  n216 = call "Inst_K2002.vi"("error in"=w4, "All Message Queues in"=w5, "Prueba31 in"=w6) -> ("error out"=w10:errorcluster)  [unwired: 8 in]
  n217 = call "Inst_CNT90.vi"("error in"=w4, "All Message Queues in"=w5, "Prueba031 in"=w6) -> ()  [unwired: 8 in, 1 out]
  n218 = Unregister For Events(event registration refnum=w21, error in=w22) -> (error out=w18:errorcluster)
  n219 = Merge Errors(w18, w17, w4, w11, w10, w8) -> (w16:errorcluster)
  n220 = disable-structure shown="Enabled" {
    frame Disabled {
      n221 = call "ingresaMediciones.vi"() -> ()  [unwired: 10 in, 2 out]
    }
    frame Enabled {
    }
  }
  n222 = call "Destroy User Event - Stop.vi"("error in (no error)"=w16, "User Event"=w14) -> ("error out"=→"error out":errorcluster)  [unwired: 9 in]
